vi "PrunePath.vi"(9 "Dest int":T1, 10 "Robot in":T3, 11 "Path in":dbl[][](array[numeric])) -> (2 "Dest out":T1, 3 "Path out":dbl[][](array[numeric]))   [LabVIEW 2018]
uses:
  Core/AI Robot.ctl
  Intel/Functions Enum.ctl
  Intel/AttackerStates.ctl
  PathDests.ctl
  PathDest.ctl
  ee49d366-d383-4f38-a751-7cc7c2738a4b.vi
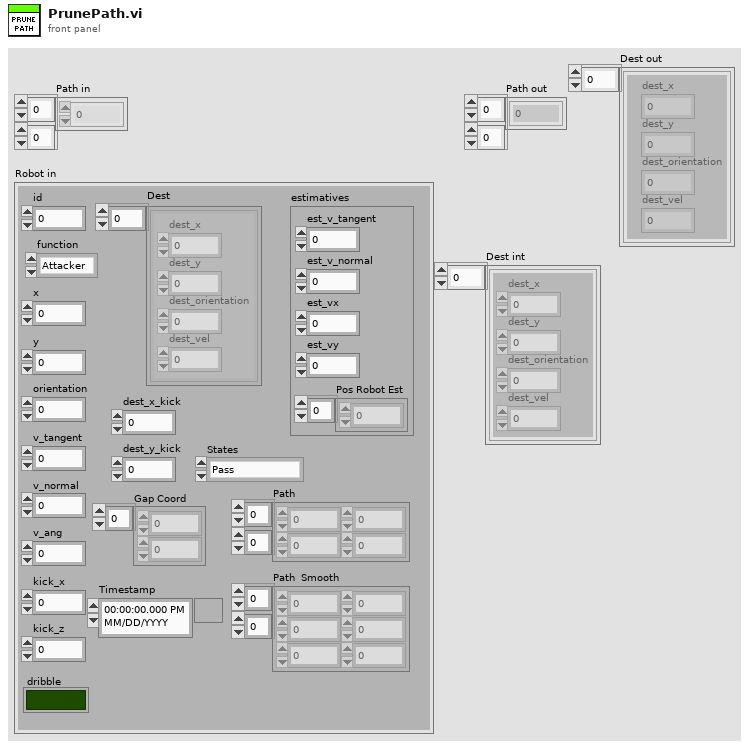
[diagram p1: front panel]
types:
  T1 = typedef "PathDests.ctl" = T2[]
  T2 = typedef "PathDest.ctl" = cluster{"dest_x":dbl, "dest_y":dbl, "dest_orientation":dbl, "dest_vel":dbl}
  T3 = typedef "AI Robot.ctl" = cluster{"id":u32, "function":T4, "x":dbl, "y":dbl, "orientation":dbl, "v_tangent":dbl, "v_normal":dbl, "v_ang":dbl, "kick_x":dbl, "kick_z":dbl, "dribble":bool, "Timestamp":timestamp, "estimatives":cluster{"est_v_tangent":dbl, "est_v_normal":dbl, "est_vx":dbl, "est_vy":dbl, "Pos Robot Est":dbl[]}, "dest_x_kick":dbl, "dest_y_kick":dbl, "Gap Coord":dbl[], "States":T5, "Path ":dbl[][], "Path  Smooth":dbl[][], "Dest":T1}
  T4 = typedef "Functions Enum.ctl" = enum16{"Attacker", "Goalie", "Defender", "Striker", "Goto 0", "Dummy", "Kicker", "ZigZag"}
  T5 = typedef "AttackerStates.ctl" = enum16{"Pass", "GoToTangent", "BallGetting", "GoToKick", "Rotate anti-clockwise", "Rotate Clockwise", ""}
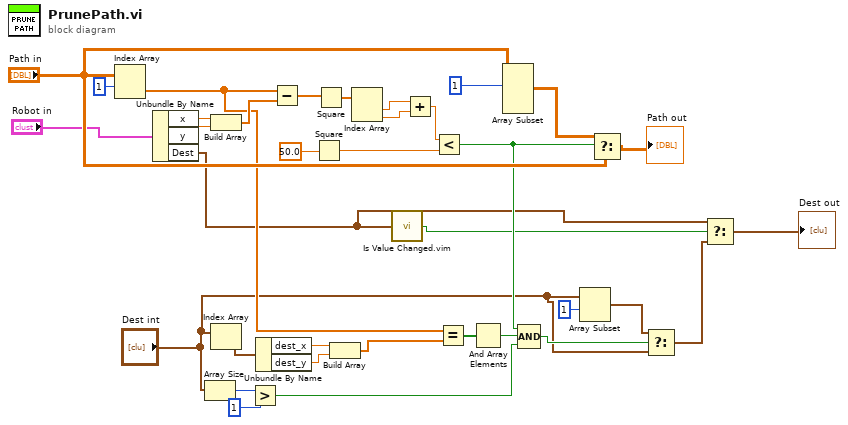
[diagram p0: block diagram]
diagram:
  n1 = Index Array(array="Path in", index (row)=1) -> (element=w19:dbl[])  [unwired: 1 in]
  n2 = Unbundle By Name("Robot in") -> ("x"=w24:dbl, "y"=w23:dbl, "Dest"=w1:T1)
  n3 = Array Size(array="Dest int") -> (size(s)=w13:i32)
  n4 = Build Array(w24, w23) -> (w25:dbl[])
  n5 = Index Array(array="Dest int") -> (element=w5:T2)  [unwired: 1 in]
  n6 = Greater?(x=w13, y=1) -> (0:w11:bool)
  n7 = Unbundle By Name(w5) -> ("dest_x"=w18:dbl, "dest_y"=w17:dbl)
  n8 = Subtract(x=w19, y=w25) -> (x-y=w26:dbl[])
  n9 = Square(x=50.0) -> (x^2=w28:dbl)
  n10 = Square(x=w26) -> (x^2=w29:dbl[])
  n11 = Build Array(w18, w17) -> (w16:dbl[])
  n12 = Index Array(array=w29) -> (element #1=w30:dbl, element #2=w31:dbl)  [unwired: 2 in]
  n13 = call "Is Value Changed.vim"("value"=w1) -> ("changed or first call?"=w4:bool)
  n14 = Add(x=w30, y=w31) -> (x+y=w32:dbl)
  n15 = Less?(x=w32, y=w28) -> (x < y?=w15:bool)
  n16 = Equal?(x=w19, y=w16) -> (x = y?=w8:bool[])
  n17 = And Array Elements(Boolean array=w8) -> (logical AND=w7:bool)
  n18 = Array Subset(array="Path in", index (row)=1 ("index")) -> (w34:dbl[][])  [unwired: 3 in]
  n19 = Compound Arithmetic op=AND(w15, w7, w11) -> (w10:bool)
  n20 = Array Subset(array="Dest int", index=1) -> (w9:T1)  [unwired: 1 in]
  n21 = Select(t=w34, s=w15, f="Path in") -> (s? t:f=→"Path out":dbl[][])
  n22 = Select(t=w9, s=w10, f="Dest int") -> (s? t:f=w3:T1)
  n23 = Select(t=w1, s=w4, f=w3) -> (s? t:f=→"Dest out":T1)
